vi "Clear Position.vi"(6 "State":T1=enum."Idle", 8 "error in (no error)":errorcluster, 11 "2DPanelBlank in":refnum<class "2DPanelBlank.lvclass">) -> (0 "error out":errorcluster, 3 "2DPanelBlank out":refnum<class "2DPanelBlank.lvclass">)   [LabVIEW 2020, in "OOPanel.lvlib" / "2DPanelBlank.lvclass"]
uses:
  2DPanelBlank.lvclass
  State.ctl
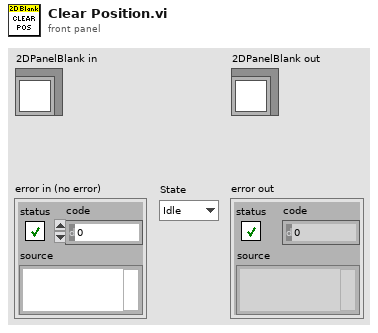
[diagram p1: front panel]
types:
  T1 = typedef "OOPanel.lvlib/2DPanelBlank.lvclass/State.ctl" = enum16{"New", "Idle", "Pool", "Used", "No SP"}
  T2 = typedef "OOPanel.lvlib/2DPanelBlank.lvclass/Info.ctl" = cluster{"Index":T3, "State":T1, "Pull Count":i32}
  T3 = typedef "OOPanel.lvlib/2D Index.ctl" = cluster{"Row":i32, "Col":i32}
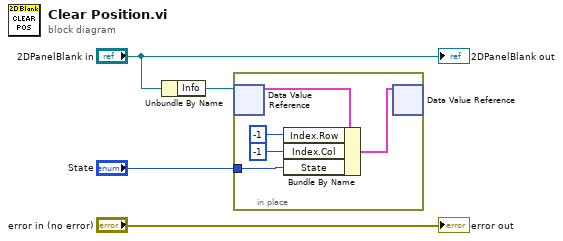
[diagram p0: block diagram]
diagram:
  n1 = Unbundle By Name("2DPanelBlank in") -> ("Info"=w3:refnum<data-value>)
  n2 = in-place {
    in-place-border: "State" -> [w5]
    n3 = in-place-dvr #1(w3) -> (w9:T2)  [unwired: 1 out]
    n4 = Bundle By Name(cluster=w9, "Index.Row"=-1 ("Row"), "Index.Col"=-1 ("Col"), "State"=w5) -> (w8:T2)
    n5 = in-place-dvr #1(w8) -> ()  [unwired: 2 out]
  }
  "error out" <- "error in (no error)"
  "2DPanelBlank out" <- "2DPanelBlank in"
